vi "OldLogToSpreadsheet.vi"() -> ()   [LabVIEW 2012]
doc: "Processes data from status data logs. Requires the user to select the date the log was taken and the log file, then runs through it and finds each time we wrote to the log, and uses the number of times we wrote as the time. It then graphs all the information that is easily graphed and useful. Other data can be obtained by finding it in the case structure in the for loop.\n\n-By Elizabeth Mahon"
uses:
  2-Think/2 Typedefs/Which Boat.ctl
  2-Think/2 Typedefs/heading.ctl
  2-Think/2 Typedefs/rate of turn.ctl
  2-Think/2 Typedefs/generalized sensor status.ctl
  2-Think/2 Typedefs/indicator LED.ctl
  2-Think/2 Typedefs/apparent wind direction.ctl
  2-Think/2 Typedefs/apparent wind speed.ctl
  2-Think/2 Typedefs/absolute wind direction.ctl
  2-Think/2 Typedefs/absolute wind speed.ctl
  0x2-OCU-Think Comm/0x2 Typedefs/Current Waypoint.ctl
  2-Think/2 Typedefs/rudder angle.ctl
  2-Think/2 Typedefs/sail setpt.ctl
  0x2-OCU-Think Comm/0x2 Typedefs/manual override.ctl
  2-Think/2 Typedefs/setpoints to boat.ctl
  <vilib>/Utility/file.llb/Write To Spreadsheet File (DBL).vi
panel:
  out "Percent Complete":u8(slide) scale=0.0..100.0
  in  "Stop early":bool
  out "Processing File....":path
  in  "Select date the log was taken":enum32{"Prior to 4/20/2012", "Post 4/20/2012"}(tab)
  in  "Data Log":T15 {"Current Waypoint Coords"."North" format="%#_10f"; "Current Waypoint Coords"."East" format="%#_8f"; "Robot Pitch/Roll"."Roll" format="%05.1f"; "Robot Pitch/Roll"."Pitch" format="%05.1f"; "Robot\nRate of Turn" format="%05.1f"; "Robot\nHeading" format="%05.1f"; "Robot UTM Location"."North" format="%#_10f"; "Robot UTM Location"."East" format="%#_8f"}
  in  "Data Log":T16 {"Current Waypoint Coords"."North" format="%#_10f"; "Current Waypoint Coords"."East" format="%#_8f"; "Robot Pitch/Roll"."Roll" format="%05.1f"; "Robot Pitch/Roll"."Pitch" format="%05.1f"; "Robot\nRate of Turn" format="%05.1f"; "Robot\nHeading" format="%05.1f"; "Robot UTM Location"."North" format="%#_10f"; "Robot UTM Location"."East" format="%#_8f"}
  # "NOTE: This has to be disconnected from the type def, because labview freaks out when the data taken != what this says it should be. Even in little things like type. So depending on how old the data is, you might need to change some things...."
  # "Where Am I?"
  # "Path Planning"
  # "From Planning Functions"
  # "(this is not a cluster because subitems\nare generated in parallel code)"
  # "NOTE:\n4/20/12 - changed from Timestamp\nto string to record time"
  # "How Am I?"
  # "What's Around Me?"
  # "As Measured"
  # "As Measured"
  # "Loop Rates"
  # "Where Am I?"
  # "Path Planning"
  # "From Planning Functions"
  # "(this is not a cluster because subitems\nare generated in parallel code)"
  # "How Am I?"
  # "What's Around Me?"
  # "As Measured"
  # "As Measured"
  # "Loop Rates"
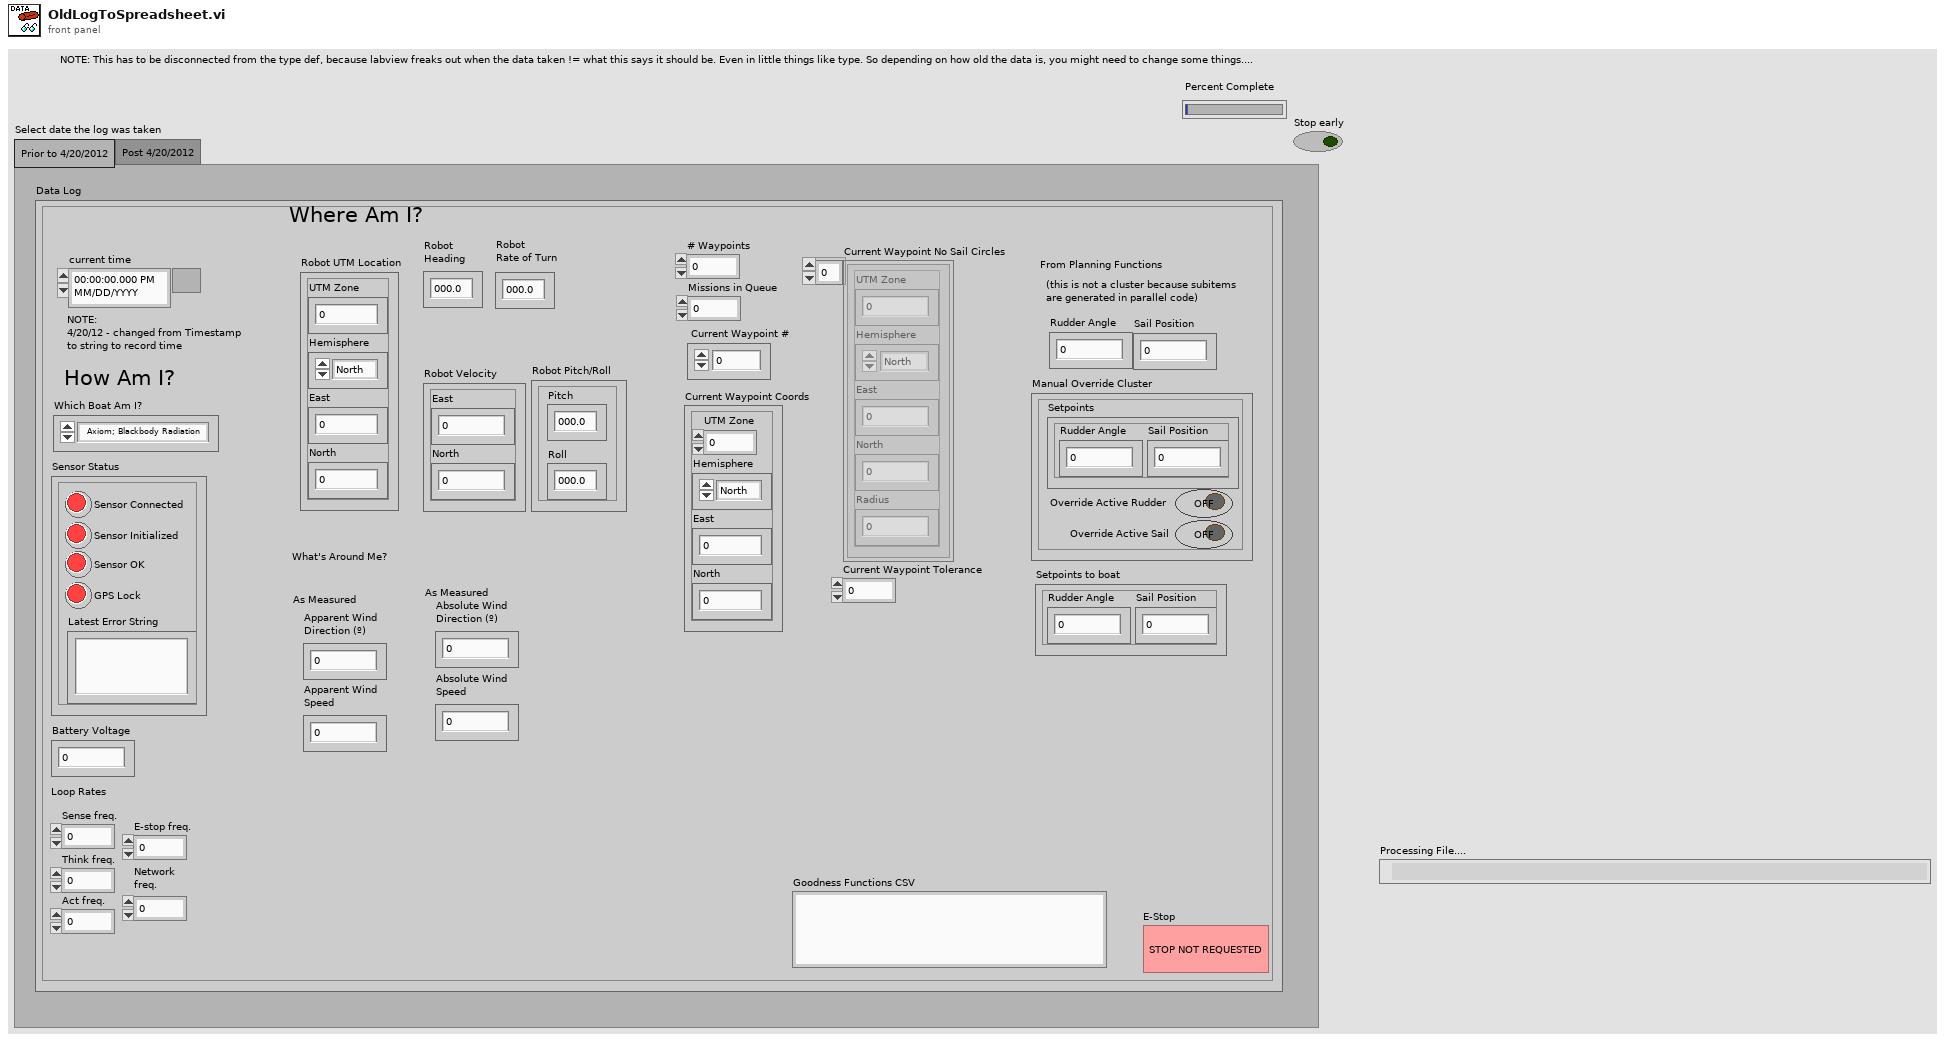
[diagram p1: front panel]
types:
  T1 = typedef "Which Boat.ctl" = enum16{"Axiom; Blackbody Radiation", "Simulation"}
  T2 = typedef "heading.ctl" = dbl
  T3 = typedef "rate of turn.ctl" = dbl
  T4 = typedef "generalized sensor status.ctl" = cluster{"Sensor Connected":T5, "Sensor Initialized":T5, "Sensor OK":T5, "Latest Error String":string, "GPS Lock":T5}
  T5 = typedef "indicator LED.ctl" = bool
  T6 = typedef "apparent wind direction.ctl" = dbl
  T7 = typedef "apparent wind speed.ctl" = dbl
  T8 = typedef "absolute wind direction.ctl" = dbl
  T9 = typedef "absolute wind speed.ctl" = dbl
  T10 = typedef "Current Waypoint.ctl" = i32
  T11 = typedef "rudder angle.ctl" = dbl
  T12 = typedef "sail setpt.ctl" = dbl
  T13 = typedef "manual override.ctl" = cluster{"Override Active Rudder":bool, "Setpoints":T14, "Override Active Sail":bool}
  T14 = typedef "setpoints to boat.ctl" = cluster{"Sail Position":T12, "Rudder Angle":T11}
  T15 = cluster{"current time":timestamp, "Which Boat Am I?":T1, "Robot UTM Location":cluster{"UTM Zone":dbl, "Hemisphere":enum16{"North", "South"}, "East":dbl, "North":dbl}, "Robot\nHeading ":T2, "Robot\nRate of Turn":T3, "Robot Velocity":cluster{"East":dbl, "North":dbl}, "Robot Pitch/Roll":cluster{"Pitch":dbl, "Roll":dbl}, "Sensor Status":T4, "Battery Voltage":dbl, "Sense freq.":dbl, "Think freq.":dbl, "Act freq.":dbl, "E-stop freq.":dbl, "Network \nfreq.":dbl, "Apparent Wind\nDirection (º)":T6, "Apparent Wind\nSpeed":T7, "Absolute Wind\nDirection (º)":T8, "Absolute Wind\nSpeed":T9, "Missions in Queue":i32, "# Waypoints":i32, " Current Waypoint #":T10, "Current Waypoint Coords":cluster{"UTM Zone":dbl, "Hemisphere":enum16{"North", "South"}, "East":dbl, "North":dbl}, "Current Waypoint Tolerance":dbl, "Current Waypoint No Sail Circles":cluster{"UTM Zone":dbl, "Hemisphere":enum16{"North", "South"}, "East":dbl, "North":dbl, "Radius":dbl}[], "Rudder Angle":T11, "Sail Position":T12, "Manual Override Cluster":T13, "Setpoints to boat":T14, "E-Stop":bool, "Goodness Functions CSV":string}
  T16 = cluster{"Which Boat Am I?":enum16{"Competition Boat", "Small RC", "Simulation"}, "Robot UTM Location":cluster{"UTM Zone":dbl, "Hemisphere":enum16{"North", "South"}, "East":dbl, "North":dbl}, "Robot\nHeading ":T2, "Robot\nRate of Turn":T3, "Robot Velocity":cluster{"East":dbl, "North":dbl}, "Robot Pitch/Roll":cluster{"Pitch":dbl, "Roll":dbl}, "Sensor Status":T4, "Battery Voltage":dbl, "Sense freq.":dbl, "Think freq.":dbl, "Act freq.":dbl, "E-stop freq.":dbl, "Network \nfreq.":dbl, "Apparent Wind\nDirection (º)":T6, "Apparent Wind\nSpeed":T7, "Absolute Wind\nDirection (º)":T8, "Absolute Wind\nSpeed":T9, "Missions in Queue":i32, "# Waypoints":i32, " Current Waypoint #":T10, "Current Waypoint Coords":cluster{"UTM Zone":dbl, "Hemisphere":enum16{"North", "South"}, "East":dbl, "North":dbl}, "Current Waypoint Tolerance":dbl, "Current Waypoint No Sail Circles":cluster{"UTM Zone":dbl, "Hemisphere":enum16{"North", "South"}, "East":dbl, "North":dbl, "Radius":dbl}[], "Rudder Angle":T11, "Sail Position":T12, "Manual Override Cluster":T13, "Setpoints to boat":T14, "E-Stop":bool, "Goodness Functions CSV":string, "Date":string, "Time":string, "Run Protect":bool}
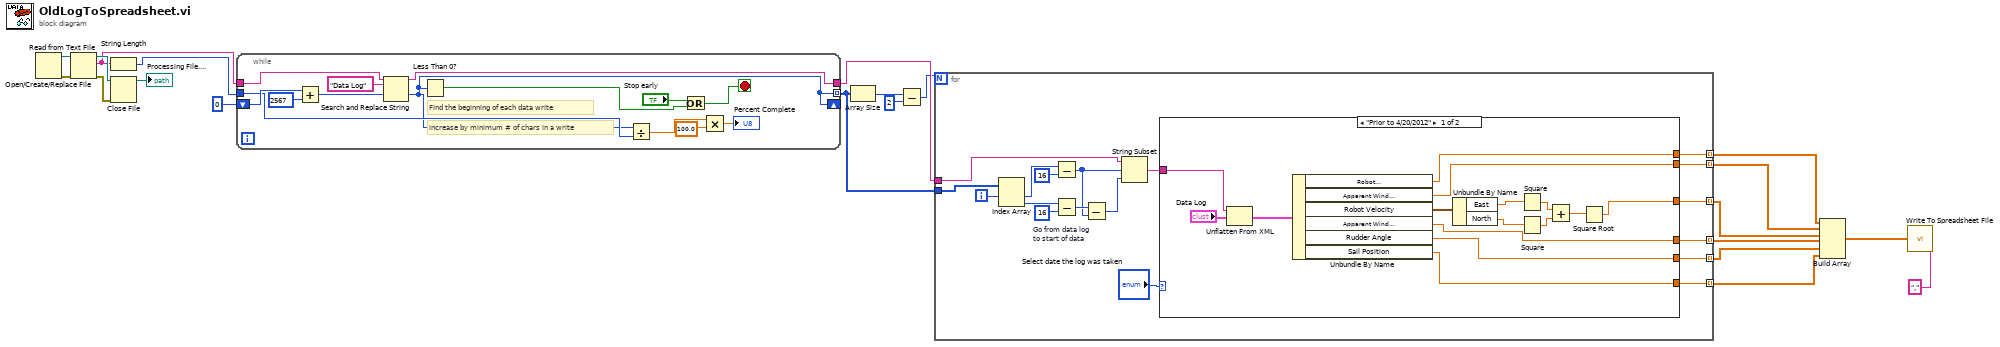
[diagram p0: block diagram]
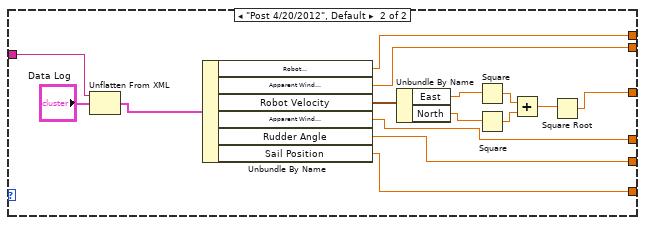
[diagram p2: hidden frame]
diagram:
  n1 = Open/Create/Replace File() -> (refnum out=w21:refnum<file>, error out=w14:errorcluster)  [unwired: 6 in, 1 out]
  n2 = Read from Text File(file (use dialog)=w21, error in=w14) -> (refnum out=w15:refnum<file>, text=w11:string, error out=w16:errorcluster)  [unwired: 2 in, 1 out]
  n3 = String Length(string=w11) -> (length=w10:i32)
  n4 = Close File(refnum=w15, error in=w16) -> (path=→"Processing File....":path)  [unwired: 1 out]
  n5 = while {
    tunnel: w11 -> [w25]
    shift-right: [w23] -> _
    shift-left: 0 ("offset past replacement") -> [w35]
    tunnel: [w24] -> w19
    tunnel: [w23] -> w12 mode=indexing
    tunnel: w10 -> [w27]
    stop <- w33 stop-if-true
    # "increase by minimum # of chars in a write"
    # "Find the beginning of each data write"
    n6 = Add(x=w35, y=2567) -> (x+y=w26:i32)
    n7 = Search and Replace String(input string=w25, search string="Data Log", offset=w26) -> (result string=w24:string, offset past replacement=w23:i32)  [unwired: 5 in, 2 out]
    n8 = Less Than 0?(x=w23) -> (x < 0?=w31:bool)
    n9 = Divide(x=w23, y=w27) -> (x/y=w30:dbl)
    n10 = Or(x="Stop early", y=w31) -> (x .or. y?=w33:bool)
    n11 = Multiply(x=w30, y=100.0) -> (x*y=→"Percent Complete":dbl)
  }
  n12 = Array Size(array=w12) -> (size(s)=w18:i32)
  n13 = Subtract(x=w18, y=2) -> (x-y=w9:i32)
  n14 = for {
    N: w9 -> [_]
    tunnel: w12 -> [w45]
    tunnel: w19 -> [w48]
    tunnel: [w41] -> w6 mode=indexing
    tunnel: [w40] -> w5 mode=indexing
    tunnel: [w39] -> w4 mode=indexing
    tunnel: [w38] -> w3 mode=indexing
    tunnel: [w37] -> w2 mode=indexing
    tunnel: [w36] -> w1 mode=indexing
    i -> [w42]
    n15 = Index Array(array=w45, index #1=w42) -> (element #1=w53:i32, element #2=w51:i32)  [unwired: 1 in]
    n16 = Subtract(x=w53, y=16) -> (x-y=w46:i32)
    n17 = Subtract "Go from data log\nto start of data"(x=w51, y=16) -> (x-y=w49:i32)
    n18 = Subtract(x=w49, y=w46) -> (x-y=w47:i32)
    n19 = String Subset(string=w48, offset (0)=w46, length (rest)=w47) -> (substring=w43:string)
    n20 = case shown="\"Prior to 4/20/2012\"" "Select date the log was taken" {
      tunnel: w43 -> [w67 w82]
      tunnel: [w58 w74] -> w41
      tunnel: [w59 w73] -> w40
      tunnel: [w57 w72] -> w39
      tunnel: [w56 w71] -> w38
      tunnel: [w55 w70] -> w37
      tunnel: [w54 w69] -> w36
      frame "Prior to 4/20/2012" {
        n21 = Unflatten From XML(xml string=w67, type="Data Log") -> (value=w60:T15)  [unwired: 1 in, 1 out]
        n22 = Unbundle By Name(w60) -> ("Robot\nHeading"=w58:T2, "Apparent Wind\nDirection (º)"=w59:T6, "Robot Velocity"=w66:cluster{"East":dbl, "North":dbl}, "Apparent Wind\nSpeed"=w56:T7, "Rudder Angle"=w55:T11, "Sail Position"=w54:T12)
        n23 = Unbundle By Name(w66) -> ("East"=w65:dbl, "North"=w64:dbl)
        n24 = Square(x=w65) -> (x^2=w62:dbl)
        n25 = Square(x=w64) -> (x^2=w63:dbl)
        n26 = Add(x=w62, y=w63) -> (x+y=w61:dbl)
        n27 = Square Root(x=w61) -> (sqrt(x)=w57:dbl)
      }
      frame "Post 4/20/2012", Default {
        n28 = Unflatten From XML(xml string=w82, type="Data Log") -> (value=w81:T16)  [unwired: 1 in, 1 out]
        n29 = Unbundle By Name(w81) -> ("Robot\nHeading"=w74:T2, "Apparent Wind\nDirection (º)"=w73:T6, "Robot Velocity"=w80:cluster{"East":dbl, "North":dbl}, "Apparent Wind\nSpeed"=w71:T7, "Rudder Angle"=w70:T11, "Sail Position"=w69:T12)
        n30 = Unbundle By Name(w80) -> ("East"=w79:dbl, "North"=w78:dbl)
        n31 = Square(x=w79) -> (x^2=w76:dbl)
        n32 = Square(x=w78) -> (x^2=w77:dbl)
        n33 = Add(x=w76, y=w77) -> (x+y=w75:dbl)
        n34 = Square Root(x=w75) -> (sqrt(x)=w72:dbl)
      }
    }
  }
  n35 = Build Array(w6, w5, w4, w3, w2, w1) -> (w8:T12[][])
  n36 = call-poly <vilib>:"Write To Spreadsheet File.vi"("delimiter (\\t)"="," ("delimiter (\\t)"), "2D data"=w8) -> ()  [unwired: 6 in, 1 out]
